vi "Emballage_BDD_bdd_initHardware.vi"(8 "error in (no error)":errorcluster) -> (0 "error out":errorcluster)   [LabVIEW 2020]
uses:
  Modules/FS/60_FS_Controles/60_FS_SetGet.ctl
  <vilib>/drjdpowell/SQLite Library/SQL Connection/Open (path).vi
  <vilib>/drjdpowell/SQLite Library/SQL Connection/Open (string).vi
  <vilib>/AdvancedString/Path To Command Line String.vi
  <vilib>/drjdpowell/SQLite Library/SQL Connection/Connection.lvclass
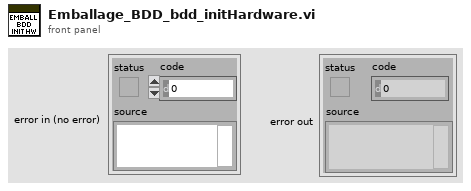
[diagram p1: front panel]
types:
  T1 = typedef "60_FS_SetGet.ctl" = enum16{"set", "get"}
  T2 = typedef "60_FS_CLT_Chemins.ctl" = cluster{"Racine_local":path, "Racine_reseau":path, "Racine_Support_Application":path, "Fichier_Journalisation":path, "Connexion_BDD_VSX":path, "Connexion_BDD_PLZ":path}
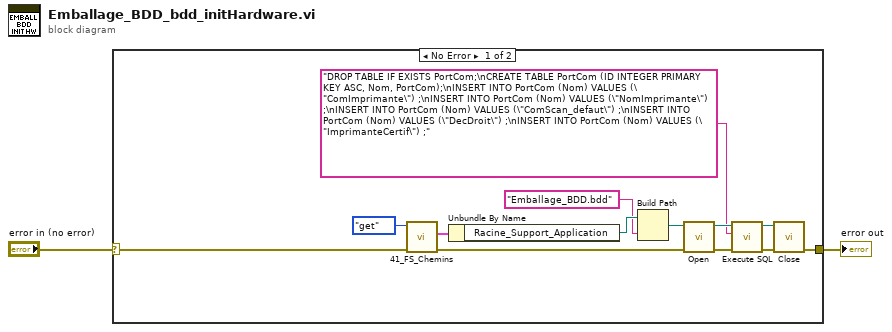
[diagram p0: block diagram]
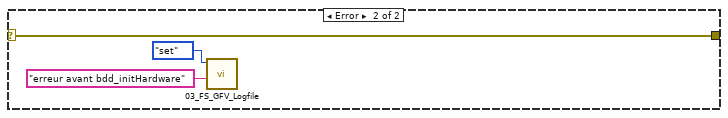
[diagram p2: hidden frame]
diagram:
  n1 = case shown="No Error" "error in (no error)" {
    selector: "error in (no error)" -> [w4 w18]
    tunnel: [w3 w18] -> w1
    frame No Error {
      n2 = call "41_FS_Chemins.vi"("error in (no error)"=w4, "SetGet"=60_FS_SetGet."get") -> ("error out"=w7:errorcluster, "CLT_Chemins_out"=w5:T2)  [unwired: 8 in]
      n3 = Unbundle By Name(w5) -> ("Racine_Support_Application"=w10:path)
      n4 = Build Path(base path=w10, name or relative path="Emballage_BDD.bdd" ("nom ou chemin relatif")) -> (appended path=w8:path)
      n5 = call-poly <vilib>:"Open.vi"("error in (no error)"=w7, "db file"=w8) -> ("error out"=w13:errorcluster, "SQLite Connection"=w15:refnum<class "Connection.lvclass">)  [unwired: 8 in]
      n6 = call <vilib>:"Execute SQL.vi"("error in (no error)"=w13, "SQL"="DROP TABLE IF EXISTS PortCom;\nCREATE TABLE PortCom (ID INTEGER PRIMARY KEY ASC, Nom, PortCom);\nINSERT INTO PortCom (Nom) VALUES (\"ComImprimante\") ;\nINSERT INTO PortCom (Nom) VALUES (\"NomImprimante\") ;\nINSERT INTO PortCom (Nom) VALUES (\"ComScan_defaut\") ;\nINSERT INTO PortCom (Nom) VALUES (\"DecDroit\") ;\nINSERT INTO PortCom (Nom) VALUES (\"ImprimanteCertif\") ;", "SQLite Connection in"=w15) -> ("error out"=w12:errorcluster, "SQLite Connection"=w14:refnum<class "Connection.lvclass">)  [unwired: 5 in, 2 out]
      n7 = call-dynamic "Close.vi"("error in (no error)"=w12, "SQLite Connection in"=w14) -> ("error out"=w3:errorcluster)  [unwired: 9 in]
    }
    frame Error {
      n8 = call "03_FS_GFV_Logfile.vi"("Chaîne"="erreur avant bdd_initHardware", "States"=60_FS_SetGet."set") -> ()  [unwired: 8 in, 2 out]
    }
  }
  "error out" <- w1
